vi "DigitalOutputs.vi"(0 "SPI_DIOEnable":u8, 1 "Digital_Outputs":u32, 2 "Digital_Output_Directions":u32) -> ()   [LabVIEW 2019]
uses:
  <vilib>/rvi/eio/common/nirviEmuTemplateMethod_errors.vi
  <vilib>/eio/EIOMethodNode/EIOMethodNode.xnode
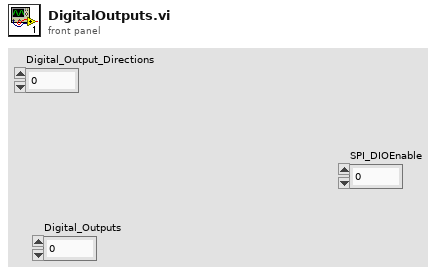
[diagram p1: front panel]
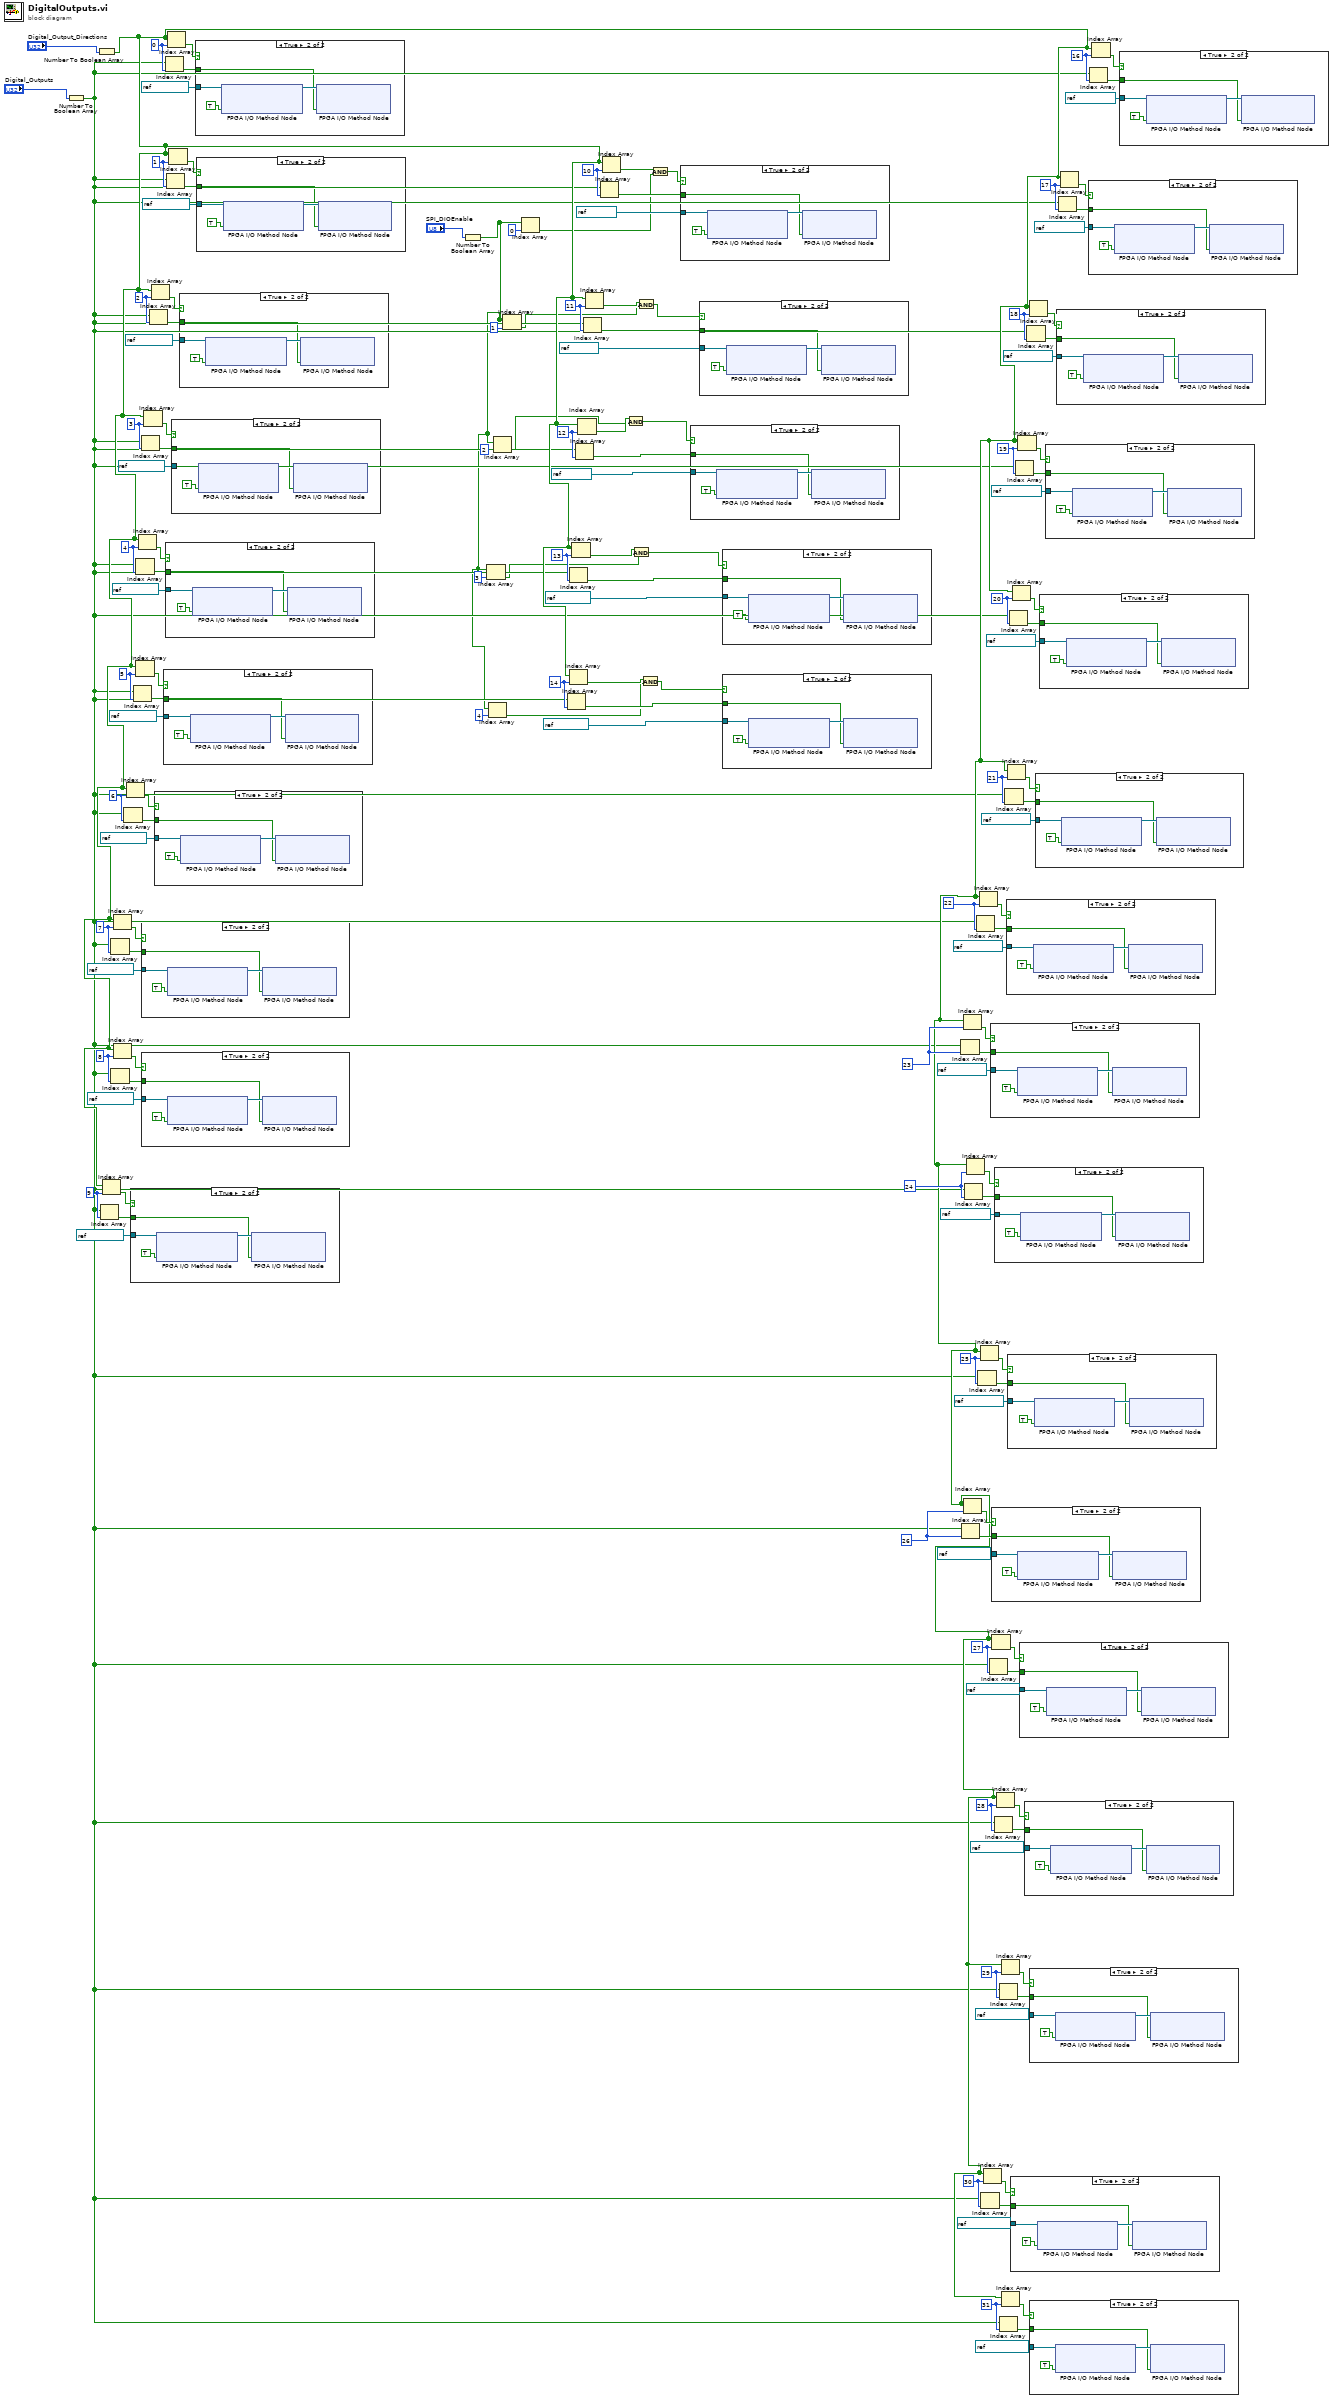
[diagram p0: block diagram]
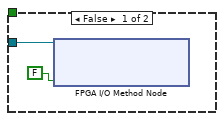
[diagram p2: hidden frame]
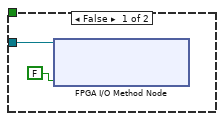
[diagram p3: hidden frame]
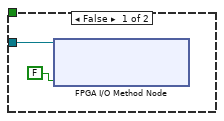
[diagram p4: hidden frame]
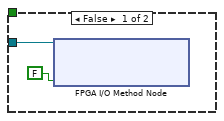
[diagram p5: hidden frame]
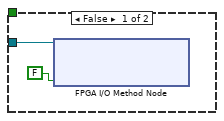
[diagram p6: hidden frame]
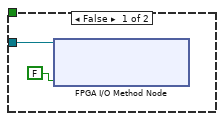
[diagram p7: hidden frame]
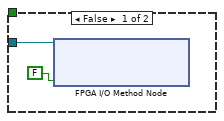
[diagram p8: hidden frame]
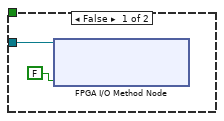
[diagram p9: hidden frame]
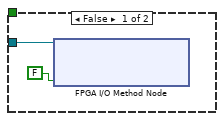
[diagram p10: hidden frame]
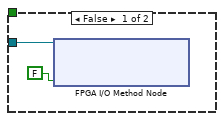
[diagram p11: hidden frame]
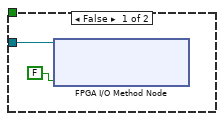
[diagram p12: hidden frame]
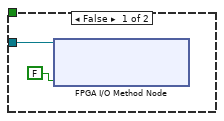
[diagram p13: hidden frame]
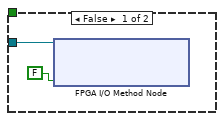
[diagram p14: hidden frame]
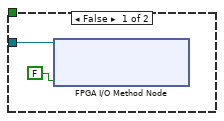
[diagram p15: hidden frame]
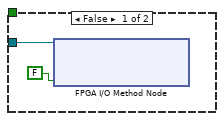
[diagram p16: hidden frame]
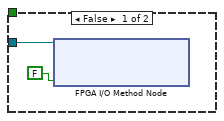
[diagram p17: hidden frame]
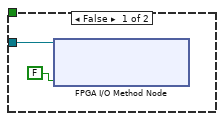
[diagram p18: hidden frame]
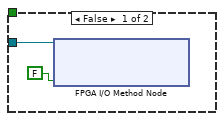
[diagram p19: hidden frame]
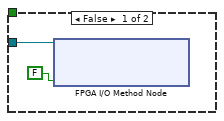
[diagram p20: hidden frame]
diagram:
  w34 = 14 ("index")
  w32 = 13 ("index")
  w30 = 12 ("index")
  w28 = 11 ("index")
  w26 = 10 ("index")
  w73 = 31 ("index")
  w75 = 30 ("index")
  w77 = 29 ("index")
  w79 = 28 ("index")
  w81 = 27 ("index")
  w83 = 26 ("index")
  w85 = 25 ("index")
  w104 = 24 ("index")
  w106 = 23 ("index")
  w108 = 22 ("index")
  w110 = 21 ("index")
  w112 = 20 ("index")
  w114 = 19 ("index")
  w116 = 18 ("index")
  w118 = 17 ("index")
  w120 = 9 ("index")
  w122 = 8 ("index")
  w124 = 7 ("index")
  w126 = 6 ("index")
  w128 = 5 ("index")
  w130 = 4 ("index")
  w132 = 3 ("index")
  w134 = 2 ("index")
  w136 = 1 ("index")
  w139 = 16 ("index")
  w141 = 0 ("index")
  n1 = Number To Boolean Array(number="Digital_Outputs") -> (Boolean array=w23:bool[])
  n2 = Number To Boolean Array(number="Digital_Output_Directions") -> (Boolean array=w24:bool[])
  n3 = Index Array(array=w23, index=w120) -> (element=w94:bool)
  n4 = Index Array(array=w24, index=w120) -> (element=w102:bool)
  n5 = Index Array(array=w23, index=w124) -> (element=w92:bool)
  n6 = Index Array(array=w23, index=w122) -> (element=w93:bool)
  n7 = Index Array(array=w24, index=w124) -> (element=w100:bool)
  n8 = Index Array(array=w24, index=w122) -> (element=w101:bool)
  n9 = Index Array(array=w23, index=w126) -> (element=w91:bool)
  n10 = Index Array(array=w24, index=w126) -> (element=w99:bool)
  n11 = case shown="True" w102 {
    tunnel: refnum<k21> "DIO/DIO9" ("FPGA I/O In") -> [w147 w151]
    tunnel: w94 -> [_ w148]
    frame False {
      n12 = xnode "FPGA I/O Method Node"("FPGA I/O In"=w147, "Enable"=FALSE) -> ()  [unwired: 1 out]
    }
    frame True {
      n13 = xnode "FPGA I/O Method Node"("FPGA I/O In"=w151, "Enable"=TRUE) -> ("FPGA I/O Out"=w149:refnum<k21>)
      n14 = xnode "FPGA I/O Method Node"("FPGA I/O In"=w149, "Data"=w148) -> ()  [unwired: 1 out]
    }
  }
  n15 = Index Array(array=w23, index=w128) -> (element=w90:bool)
  n16 = Index Array(array=w23, index=w130) -> (element=w89:bool)
  n17 = Index Array(array=w24, index=w128) -> (element=w98:bool)
  n18 = Index Array(array=w24, index=w130) -> (element=w97:bool)
  n19 = case shown="True" w100 {
    tunnel: refnum<k21> "DIO/DIO7" ("FPGA I/O In") -> [w153 w157]
    tunnel: w92 -> [_ w154]
    frame False {
      n20 = xnode "FPGA I/O Method Node"("FPGA I/O In"=w153, "Enable"=FALSE) -> ()  [unwired: 1 out]
    }
    frame True {
      n21 = xnode "FPGA I/O Method Node"("FPGA I/O In"=w157, "Enable"=TRUE) -> ("FPGA I/O Out"=w155:refnum<k21>)
      n22 = xnode "FPGA I/O Method Node"("FPGA I/O In"=w155, "Data"=w154) -> ()  [unwired: 1 out]
    }
  }
  n23 = case shown="True" w101 {
    tunnel: refnum<k21> "DIO/DIO8" ("FPGA I/O In") -> [w159 w163]
    tunnel: w93 -> [_ w160]
    frame False {
      n24 = xnode "FPGA I/O Method Node"("FPGA I/O In"=w159, "Enable"=FALSE) -> ()  [unwired: 1 out]
    }
    frame True {
      n25 = xnode "FPGA I/O Method Node"("FPGA I/O In"=w163, "Enable"=TRUE) -> ("FPGA I/O Out"=w161:refnum<k21>)
      n26 = xnode "FPGA I/O Method Node"("FPGA I/O In"=w161, "Data"=w160) -> ()  [unwired: 1 out]
    }
  }
  n27 = Index Array(array=w23, index=w132) -> (element=w88:bool)
  n28 = Index Array(array=w24, index=w132) -> (element=w96:bool)
  n29 = Index Array(array=w23, index=w134) -> (element=w87:bool)
  n30 = Index Array(array=w24, index=w134) -> (element=w95:bool)
  n31 = case shown="True" w99 {
    tunnel: refnum<k21> "DIO/DIO6" ("FPGA I/O In") -> [w165 w169]
    tunnel: w91 -> [_ w166]
    frame False {
      n32 = xnode "FPGA I/O Method Node"("FPGA I/O In"=w165, "Enable"=FALSE) -> ()  [unwired: 1 out]
    }
    frame True {
      n33 = xnode "FPGA I/O Method Node"("FPGA I/O In"=w169, "Enable"=TRUE) -> ("FPGA I/O Out"=w167:refnum<k21>)
      n34 = xnode "FPGA I/O Method Node"("FPGA I/O In"=w167, "Data"=w166) -> ()  [unwired: 1 out]
    }
  }
  n35 = case shown="True" w98 {
    tunnel: refnum<k21> "DIO/DIO5" ("FPGA I/O In") -> [w171 w175]
    tunnel: w90 -> [_ w172]
    frame False {
      n36 = xnode "FPGA I/O Method Node"("FPGA I/O In"=w171, "Enable"=FALSE) -> ()  [unwired: 1 out]
    }
    frame True {
      n37 = xnode "FPGA I/O Method Node"("FPGA I/O In"=w175, "Enable"=TRUE) -> ("FPGA I/O Out"=w173:refnum<k21>)
      n38 = xnode "FPGA I/O Method Node"("FPGA I/O In"=w173, "Data"=w172) -> ()  [unwired: 1 out]
    }
  }
  n39 = Index Array(array=w23, index=w141) -> (element=w40:bool)
  n40 = case shown="True" w97 {
    tunnel: refnum<k21> "DIO/DIO4" ("FPGA I/O In") -> [w177 w181]
    tunnel: w89 -> [_ w178]
    frame False {
      n41 = xnode "FPGA I/O Method Node"("FPGA I/O In"=w177, "Enable"=FALSE) -> ()  [unwired: 1 out]
    }
    frame True {
      n42 = xnode "FPGA I/O Method Node"("FPGA I/O In"=w181, "Enable"=TRUE) -> ("FPGA I/O Out"=w179:refnum<k21>)
      n43 = xnode "FPGA I/O Method Node"("FPGA I/O In"=w179, "Data"=w178) -> ()  [unwired: 1 out]
    }
  }
  n44 = Index Array(array=w23, index=w136) -> (element=w103:bool)
  n45 = Index Array(array=w24, index=w141) -> (element=w143:bool)
  n46 = Index Array(array=w24, index=w136) -> (element=w138:bool)
  n47 = case shown="True" w96 {
    tunnel: refnum<k21> "DIO/DIO3" ("FPGA I/O In") -> [w183 w187]
    tunnel: w88 -> [_ w184]
    frame False {
      n48 = xnode "FPGA I/O Method Node"("FPGA I/O In"=w183, "Enable"=FALSE) -> ()  [unwired: 1 out]
    }
    frame True {
      n49 = xnode "FPGA I/O Method Node"("FPGA I/O In"=w187, "Enable"=TRUE) -> ("FPGA I/O Out"=w185:refnum<k21>)
      n50 = xnode "FPGA I/O Method Node"("FPGA I/O In"=w185, "Data"=w184) -> ()  [unwired: 1 out]
    }
  }
  n51 = case shown="True" w95 {
    tunnel: refnum<k21> "DIO/DIO2" ("FPGA I/O In") -> [w189 w193]
    tunnel: w87 -> [_ w190]
    frame False {
      n52 = xnode "FPGA I/O Method Node"("FPGA I/O In"=w189, "Enable"=FALSE) -> ()  [unwired: 1 out]
    }
    frame True {
      n53 = xnode "FPGA I/O Method Node"("FPGA I/O In"=w193, "Enable"=TRUE) -> ("FPGA I/O Out"=w191:refnum<k21>)
      n54 = xnode "FPGA I/O Method Node"("FPGA I/O In"=w191, "Data"=w190) -> ()  [unwired: 1 out]
    }
  }
  n55 = case shown="True" w143 {
    tunnel: refnum<k21> "DIO/DIO0" ("FPGA I/O In") -> [w195 w199]
    tunnel: w40 -> [_ w196]
    frame False {
      n56 = xnode "FPGA I/O Method Node"("FPGA I/O In"=w195, "Enable"=FALSE) -> ()  [unwired: 1 out]
    }
    frame True {
      n57 = xnode "FPGA I/O Method Node"("FPGA I/O In"=w199, "Enable"=TRUE) -> ("FPGA I/O Out"=w197:refnum<k21>)
      n58 = xnode "FPGA I/O Method Node"("FPGA I/O In"=w197, "Data"=w196) -> ()  [unwired: 1 out]
    }
  }
  n59 = case shown="True" w138 {
    tunnel: refnum<k21> "DIO/DIO1" ("FPGA I/O In") -> [w201 w205]
    tunnel: w103 -> [_ w202]
    frame False {
      n60 = xnode "FPGA I/O Method Node"("FPGA I/O In"=w201, "Enable"=FALSE) -> ()  [unwired: 1 out]
    }
    frame True {
      n61 = xnode "FPGA I/O Method Node"("FPGA I/O In"=w205, "Enable"=TRUE) -> ("FPGA I/O Out"=w203:refnum<k21>)
      n62 = xnode "FPGA I/O Method Node"("FPGA I/O In"=w203, "Data"=w202) -> ()  [unwired: 1 out]
    }
  }
  n63 = Number To Boolean Array(number="SPI_DIOEnable") -> (Boolean array=w13:bool[])
  n64 = Index Array(array=w13, index=3) -> (element=w3:bool)
  n65 = Index Array(array=w13, index=4) -> (element=w11:bool)
  n66 = Index Array(array=w13, index=2) -> (element=w5:bool)
  n67 = Index Array(array=w13, index=1) -> (element=w8:bool)
  n68 = Index Array(array=w13, index=0) -> (element=w19:bool)
  n69 = Index Array(array=w23, index=w34) -> (element=w36:bool)
  n70 = Index Array(array=w23, index=w32) -> (element=w37:bool)
  n71 = Index Array(array=w24, index=w34) -> (element=w12:bool)
  n72 = Index Array(array=w24, index=w32) -> (element=w4:bool)
  n73 = Index Array(array=w23, index=w30) -> (element=w38:bool)
  n74 = Index Array(array=w24, index=w30) -> (element=w6:bool)
  n75 = Index Array(array=w23, index=w28) -> (element=w39:bool)
  n76 = Index Array(array=w24, index=w28) -> (element=w9:bool)
  n77 = Index Array(array=w23, index=w26) -> (element=w35:bool)
  n78 = Index Array(array=w24, index=w26) -> (element=w20:bool)
  n79 = And(x=w6, y=w5) -> (x .and. y?=w1:bool)
  n80 = And(x=w4, y=w3) -> (x .and. y?=w2:bool)
  n81 = And(x=w9, y=w8) -> (x .and. y?=w7:bool)
  n82 = And(x=w12, y=w11) -> (x .and. y?=w10:bool)
  n83 = And(x=w20, y=w19) -> (x .and. y?=w18:bool)
  n84 = case shown="True" w18 {
    tunnel: refnum<k21> "SPI CS1" ("FPGA I/O In") -> [w207 w211]
    tunnel: w35 -> [_ w208]
    frame False {
      n85 = xnode "FPGA I/O Method Node"("FPGA I/O In"=w207, "Enable"=FALSE) -> ()  [unwired: 1 out]
    }
    frame True {
      n86 = xnode "FPGA I/O Method Node"("FPGA I/O In"=w211, "Enable"=TRUE) -> ("FPGA I/O Out"=w209:refnum<k21>)
      n87 = xnode "FPGA I/O Method Node"("FPGA I/O In"=w209, "Data"=w208) -> ()  [unwired: 1 out]
    }
  }
  n88 = case shown="True" w1 {
    tunnel: refnum<k21> "SPI CS3" ("FPGA I/O In") -> [w213 w217]
    tunnel: w38 -> [_ w214]
    frame False {
      n89 = xnode "FPGA I/O Method Node"("FPGA I/O In"=w213, "Enable"=FALSE) -> ()  [unwired: 1 out]
    }
    frame True {
      n90 = xnode "FPGA I/O Method Node"("FPGA I/O In"=w217, "Enable"=TRUE) -> ("FPGA I/O Out"=w215:refnum<k21>)
      n91 = xnode "FPGA I/O Method Node"("FPGA I/O In"=w215, "Data"=w214) -> ()  [unwired: 1 out]
    }
  }
  n92 = case shown="True" w7 {
    tunnel: refnum<k21> "SPI CS2" ("FPGA I/O In") -> [w219 w223]
    tunnel: w39 -> [_ w220]
    frame False {
      n93 = xnode "FPGA I/O Method Node"("FPGA I/O In"=w219, "Enable"=FALSE) -> ()  [unwired: 1 out]
    }
    frame True {
      n94 = xnode "FPGA I/O Method Node"("FPGA I/O In"=w223, "Enable"=TRUE) -> ("FPGA I/O Out"=w221:refnum<k21>)
      n95 = xnode "FPGA I/O Method Node"("FPGA I/O In"=w221, "Data"=w220) -> ()  [unwired: 1 out]
    }
  }
  n96 = case shown="True" w2 {
    tunnel: refnum<k21> "SPI MISO" ("FPGA I/O In") -> [w225 w229]
    tunnel: w37 -> [_ w226]
    frame False {
      n97 = xnode "FPGA I/O Method Node"("FPGA I/O In"=w225, "Enable"=FALSE) -> ()  [unwired: 1 out]
    }
    frame True {
      n98 = xnode "FPGA I/O Method Node"("FPGA I/O In"=w229, "Enable"=TRUE) -> ("FPGA I/O Out"=w227:refnum<k21>)
      n99 = xnode "FPGA I/O Method Node"("FPGA I/O In"=w227, "Data"=w226) -> ()  [unwired: 1 out]
    }
  }
  n100 = case shown="True" w10 {
    tunnel: refnum<k21> "SPI MISO" ("FPGA I/O In") -> [w231 w235]
    tunnel: w36 -> [_ w232]
    frame False {
      n101 = xnode "FPGA I/O Method Node"("FPGA I/O In"=w231, "Enable"=FALSE) -> ()  [unwired: 1 out]
    }
    frame True {
      n102 = xnode "FPGA I/O Method Node"("FPGA I/O In"=w235, "Enable"=TRUE) -> ("FPGA I/O Out"=w233:refnum<k21>)
      n103 = xnode "FPGA I/O Method Node"("FPGA I/O In"=w233, "Data"=w232) -> ()  [unwired: 1 out]
    }
  }
  n104 = Index Array(array=w23, index=w106) -> (element=w55:bool)
  n105 = Index Array(array=w23, index=w83) -> (element=w61:bool)
  n106 = Index Array(array=w24, index=w106) -> (element=w56:bool)
  n107 = Index Array(array=w24, index=w83) -> (element=w62:bool)
  n108 = Index Array(array=w23, index=w104) -> (element=w57:bool)
  n109 = Index Array(array=w24, index=w104) -> (element=w58:bool)
  n110 = Index Array(array=w23, index=w108) -> (element=w53:bool)
  n111 = Index Array(array=w23, index=w85) -> (element=w59:bool)
  n112 = Index Array(array=w24, index=w108) -> (element=w54:bool)
  n113 = Index Array(array=w24, index=w85) -> (element=w60:bool)
  n114 = Index Array(array=w23, index=w75) -> (element=w69:bool)
  n115 = Index Array(array=w24, index=w75) -> (element=w70:bool)
  n116 = Index Array(array=w23, index=w81) -> (element=w63:bool)
  n117 = case shown="True" w56 {
    tunnel: refnum<k21> "MXP/DIO7" ("FPGA I/O In") -> [w237 w241]
    tunnel: w55 -> [_ w238]
    frame False {
      n118 = xnode "FPGA I/O Method Node"("FPGA I/O In"=w237, "Enable"=FALSE) -> ()  [unwired: 1 out]
    }
    frame True {
      n119 = xnode "FPGA I/O Method Node"("FPGA I/O In"=w241, "Enable"=TRUE) -> ("FPGA I/O Out"=w239:refnum<k21>)
      n120 = xnode "FPGA I/O Method Node"("FPGA I/O In"=w239, "Data"=w238) -> ()  [unwired: 1 out]
    }
  }
  n121 = case shown="True" w62 {
    tunnel: refnum<k21> "MXP/DIO10" ("FPGA I/O In") -> [w243 w247]
    tunnel: w61 -> [_ w244]
    frame False {
      n122 = xnode "FPGA I/O Method Node"("FPGA I/O In"=w243, "Enable"=FALSE) -> ()  [unwired: 1 out]
    }
    frame True {
      n123 = xnode "FPGA I/O Method Node"("FPGA I/O In"=w247, "Enable"=TRUE) -> ("FPGA I/O Out"=w245:refnum<k21>)
      n124 = xnode "FPGA I/O Method Node"("FPGA I/O In"=w245, "Data"=w244) -> ()  [unwired: 1 out]
    }
  }
  n125 = Index Array(array=w24, index=w81) -> (element=w64:bool)
  n126 = case shown="True" w58 {
    tunnel: refnum<k21> "MXP/DIO8" ("FPGA I/O In") -> [w249 w253]
    tunnel: w57 -> [_ w250]
    frame False {
      n127 = xnode "FPGA I/O Method Node"("FPGA I/O In"=w249, "Enable"=FALSE) -> ()  [unwired: 1 out]
    }
    frame True {
      n128 = xnode "FPGA I/O Method Node"("FPGA I/O In"=w253, "Enable"=TRUE) -> ("FPGA I/O Out"=w251:refnum<k21>)
      n129 = xnode "FPGA I/O Method Node"("FPGA I/O In"=w251, "Data"=w250) -> ()  [unwired: 1 out]
    }
  }
  n130 = Index Array(array=w23, index=w79) -> (element=w66:bool)
  n131 = Index Array(array=w24, index=w79) -> (element=w65:bool)
  n132 = Index Array(array=w23, index=w77) -> (element=w68:bool)
  n133 = Index Array(array=w23, index=w73) -> (element=w71:bool)
  n134 = Index Array(array=w24, index=w77) -> (element=w67:bool)
  n135 = Index Array(array=w24, index=w73) -> (element=w72:bool)
  n136 = Index Array(array=w23, index=w110) -> (element=w51:bool)
  n137 = case shown="True" w54 {
    tunnel: refnum<k21> "MXP/DIO6" ("FPGA I/O In") -> [w255 w259]
    tunnel: w53 -> [_ w256]
    frame False {
      n138 = xnode "FPGA I/O Method Node"("FPGA I/O In"=w255, "Enable"=FALSE) -> ()  [unwired: 1 out]
    }
    frame True {
      n139 = xnode "FPGA I/O Method Node"("FPGA I/O In"=w259, "Enable"=TRUE) -> ("FPGA I/O Out"=w257:refnum<k21>)
      n140 = xnode "FPGA I/O Method Node"("FPGA I/O In"=w257, "Data"=w256) -> ()  [unwired: 1 out]
    }
  }
  n141 = Index Array(array=w24, index=w110) -> (element=w52:bool)
  n142 = case shown="True" w60 {
    tunnel: refnum<k21> "MXP/DIO9" ("FPGA I/O In") -> [w261 w265]
    tunnel: w59 -> [_ w262]
    frame False {
      n143 = xnode "FPGA I/O Method Node"("FPGA I/O In"=w261, "Enable"=FALSE) -> ()  [unwired: 1 out]
    }
    frame True {
      n144 = xnode "FPGA I/O Method Node"("FPGA I/O In"=w265, "Enable"=TRUE) -> ("FPGA I/O Out"=w263:refnum<k21>)
      n145 = xnode "FPGA I/O Method Node"("FPGA I/O In"=w263, "Data"=w262) -> ()  [unwired: 1 out]
    }
  }
  n146 = Index Array(array=w23, index=w112) -> (element=w50:bool)
  n147 = case shown="True" w70 {
    tunnel: refnum<k21> "MXP/DIO14" ("FPGA I/O In") -> [w267 w271]
    tunnel: w69 -> [_ w268]
    frame False {
      n148 = xnode "FPGA I/O Method Node"("FPGA I/O In"=w267, "Enable"=FALSE) -> ()  [unwired: 1 out]
    }
    frame True {
      n149 = xnode "FPGA I/O Method Node"("FPGA I/O In"=w271, "Enable"=TRUE) -> ("FPGA I/O Out"=w269:refnum<k21>)
      n150 = xnode "FPGA I/O Method Node"("FPGA I/O In"=w269, "Data"=w268) -> ()  [unwired: 1 out]
    }
  }
  n151 = Index Array(array=w24, index=w112) -> (element=w49:bool)
  n152 = Index Array(array=w23, index=w114) -> (element=w47:bool)
  n153 = Index Array(array=w24, index=w114) -> (element=w48:bool)
  n154 = case shown="True" w64 {
    tunnel: refnum<k21> "MXP/DIO11" ("FPGA I/O In") -> [w273 w277]
    tunnel: w63 -> [_ w274]
    frame False {
      n155 = xnode "FPGA I/O Method Node"("FPGA I/O In"=w273, "Enable"=FALSE) -> ()  [unwired: 1 out]
    }
    frame True {
      n156 = xnode "FPGA I/O Method Node"("FPGA I/O In"=w277, "Enable"=TRUE) -> ("FPGA I/O Out"=w275:refnum<k21>)
      n157 = xnode "FPGA I/O Method Node"("FPGA I/O In"=w275, "Data"=w274) -> ()  [unwired: 1 out]
    }
  }
  n158 = case shown="True" w65 {
    tunnel: refnum<k21> "MXP/DIO12" ("FPGA I/O In") -> [w279 w283]
    tunnel: w66 -> [_ w280]
    frame False {
      n159 = xnode "FPGA I/O Method Node"("FPGA I/O In"=w279, "Enable"=FALSE) -> ()  [unwired: 1 out]
    }
    frame True {
      n160 = xnode "FPGA I/O Method Node"("FPGA I/O In"=w283, "Enable"=TRUE) -> ("FPGA I/O Out"=w281:refnum<k21>)
      n161 = xnode "FPGA I/O Method Node"("FPGA I/O In"=w281, "Data"=w280) -> ()  [unwired: 1 out]
    }
  }
  n162 = Index Array(array=w23, index=w116) -> (element=w46:bool)
  n163 = Index Array(array=w24, index=w116) -> (element=w45:bool)
  n164 = case shown="True" w67 {
    tunnel: refnum<k21> "MXP/DIO13" ("FPGA I/O In") -> [w285 w289]
    tunnel: w68 -> [_ w286]
    frame False {
      n165 = xnode "FPGA I/O Method Node"("FPGA I/O In"=w285, "Enable"=FALSE) -> ()  [unwired: 1 out]
    }
    frame True {
      n166 = xnode "FPGA I/O Method Node"("FPGA I/O In"=w289, "Enable"=TRUE) -> ("FPGA I/O Out"=w287:refnum<k21>)
      n167 = xnode "FPGA I/O Method Node"("FPGA I/O In"=w287, "Data"=w286) -> ()  [unwired: 1 out]
    }
  }
  n168 = case shown="True" w72 {
    tunnel: refnum<k21> "MXP/DIO15" ("FPGA I/O In") -> [w291 w295]
    tunnel: w71 -> [_ w292]
    frame False {
      n169 = xnode "FPGA I/O Method Node"("FPGA I/O In"=w291, "Enable"=FALSE) -> ()  [unwired: 1 out]
    }
    frame True {
      n170 = xnode "FPGA I/O Method Node"("FPGA I/O In"=w295, "Enable"=TRUE) -> ("FPGA I/O Out"=w293:refnum<k21>)
      n171 = xnode "FPGA I/O Method Node"("FPGA I/O In"=w293, "Data"=w292) -> ()  [unwired: 1 out]
    }
  }
  n172 = case shown="True" w52 {
    tunnel: refnum<k21> "MXP/DIO5" ("FPGA I/O In") -> [w297 w301]
    tunnel: w51 -> [_ w298]
    frame False {
      n173 = xnode "FPGA I/O Method Node"("FPGA I/O In"=w297, "Enable"=FALSE) -> ()  [unwired: 1 out]
    }
    frame True {
      n174 = xnode "FPGA I/O Method Node"("FPGA I/O In"=w301, "Enable"=TRUE) -> ("FPGA I/O Out"=w299:refnum<k21>)
      n175 = xnode "FPGA I/O Method Node"("FPGA I/O In"=w299, "Data"=w298) -> ()  [unwired: 1 out]
    }
  }
  n176 = case shown="True" w49 {
    tunnel: refnum<k21> "MXP/DIO4" ("FPGA I/O In") -> [w303 w307]
    tunnel: w50 -> [_ w304]
    frame False {
      n177 = xnode "FPGA I/O Method Node"("FPGA I/O In"=w303, "Enable"=FALSE) -> ()  [unwired: 1 out]
    }
    frame True {
      n178 = xnode "FPGA I/O Method Node"("FPGA I/O In"=w307, "Enable"=TRUE) -> ("FPGA I/O Out"=w305:refnum<k21>)
      n179 = xnode "FPGA I/O Method Node"("FPGA I/O In"=w305, "Data"=w304) -> ()  [unwired: 1 out]
    }
  }
  n180 = case shown="True" w48 {
    tunnel: refnum<k21> "MXP/DIO3" ("FPGA I/O In") -> [w309 w313]
    tunnel: w47 -> [_ w310]
    frame False {
      n181 = xnode "FPGA I/O Method Node"("FPGA I/O In"=w309, "Enable"=FALSE) -> ()  [unwired: 1 out]
    }
    frame True {
      n182 = xnode "FPGA I/O Method Node"("FPGA I/O In"=w313, "Enable"=TRUE) -> ("FPGA I/O Out"=w311:refnum<k21>)
      n183 = xnode "FPGA I/O Method Node"("FPGA I/O In"=w311, "Data"=w310) -> ()  [unwired: 1 out]
    }
  }
  n184 = case shown="True" w45 {
    tunnel: refnum<k21> "MXP/DIO2" ("FPGA I/O In") -> [w315 w319]
    tunnel: w46 -> [_ w316]
    frame False {
      n185 = xnode "FPGA I/O Method Node"("FPGA I/O In"=w315, "Enable"=FALSE) -> ()  [unwired: 1 out]
    }
    frame True {
      n186 = xnode "FPGA I/O Method Node"("FPGA I/O In"=w319, "Enable"=TRUE) -> ("FPGA I/O Out"=w317:refnum<k21>)
      n187 = xnode "FPGA I/O Method Node"("FPGA I/O In"=w317, "Data"=w316) -> ()  [unwired: 1 out]
    }
  }
  n188 = Index Array(array=w23, index=w118) -> (element=w43:bool)
  n189 = Index Array(array=w24, index=w118) -> (element=w44:bool)
  n190 = case shown="True" w44 {
    tunnel: refnum<k21> "MXP/DIO1" ("FPGA I/O In") -> [w321 w325]
    tunnel: w43 -> [_ w322]
    frame False {
      n191 = xnode "FPGA I/O Method Node"("FPGA I/O In"=w321, "Enable"=FALSE) -> ()  [unwired: 1 out]
    }
    frame True {
      n192 = xnode "FPGA I/O Method Node"("FPGA I/O In"=w325, "Enable"=TRUE) -> ("FPGA I/O Out"=w323:refnum<k21>)
      n193 = xnode "FPGA I/O Method Node"("FPGA I/O In"=w323, "Data"=w322) -> ()  [unwired: 1 out]
    }
  }
  n194 = Index Array(array=w23, index=w139) -> (element=w41:bool)
  n195 = Index Array(array=w24, index=w139) -> (element=w42:bool)
  n196 = case shown="True" w42 {
    tunnel: refnum<k21> "MXP/DIO0" ("FPGA I/O In") -> [w327 w331]
    tunnel: w41 -> [_ w328]
    frame False {
      n197 = xnode "FPGA I/O Method Node"("FPGA I/O In"=w327, "Enable"=FALSE) -> ()  [unwired: 1 out]
    }
    frame True {
      n198 = xnode "FPGA I/O Method Node"("FPGA I/O In"=w331, "Enable"=TRUE) -> ("FPGA I/O Out"=w329:refnum<k21>)
      n199 = xnode "FPGA I/O Method Node"("FPGA I/O In"=w329, "Data"=w328) -> ()  [unwired: 1 out]
    }
  }
